vi "Fire Size Event.vi"(8 "error in (no error)":errorcluster, 10 "Size":T1, 11 "Terminal in":refnum<class "Terminal.lvclass">) -> (0 "error out":errorcluster, 3 "Terminal out":refnum<class "Terminal.lvclass">)   [LabVIEW 2020, in "Terminal.lvlib" / "Terminal.lvclass"]
uses:
  Terminal.lvclass
  Terminal.lvclass/Terminal.ctl
  <vilib>/Utility/miscctls.llb/LVBoundsTypeDef.ctl
  Size Event Data.ctl
  Terminal.lvlib
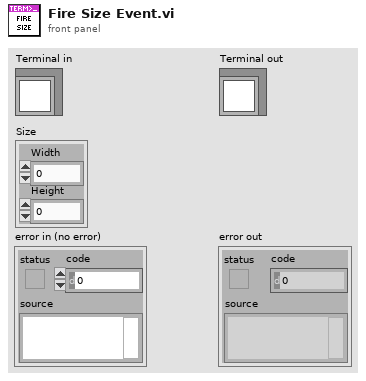
[diagram p1: front panel]
types:
  T1 = typedef "LVBoundsTypeDef.ctl" = cluster{"Width":u32, "Height":u32}
  T2 = typedef "Terminal.lvlib/Size Event Data.ctl" = cluster{"Size":T1}
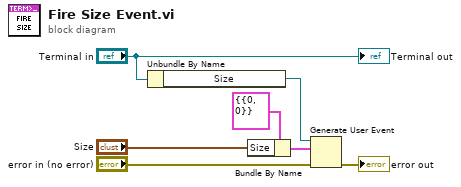
[diagram p0: block diagram]
diagram:
  n1 = Unbundle By Name("Terminal in") -> ("Size"=w6:refnum<user-event>)
  n2 = Bundle By Name(cluster=T2 {"Size"={"Width"=0, "Height"=0}} ("event data"), "Size"="Size") -> (w4:T2)
  n3 = Generate User Event(user event=w6, event data cluster=w4, error in="error in (no error)") -> (error out=→"error out":errorcluster)  [unwired: 1 in, 1 out]
  "Terminal out" <- "Terminal in"
